vi "_debug_path_create.vi"(9 "Points":T1[](array[typedef]) {"RotationTarget"."rotation"."SIN" format="%13.4f"; "RotationTarget"."rotation"."COS" format="%13.4f"; "RotationTarget"."rotation"."VALUE" format="%13.4f"; "Position"."Y" format="%14.3f"; "Position"."X" format="%14.3f"}, 11 "file path":path) -> (1 "out Points":T1[](array[typedef]) {"RotationTarget"."rotation"."SIN" format="%13.4f"; "RotationTarget"."rotation"."COS" format="%13.4f"; "RotationTarget"."rotation"."VALUE" format="%13.4f"; "Position"."Y" format="%14.3f"; "Position"."X" format="%14.3f"})   [LabVIEW 2019]
uses:
  <vilib>/Rock Robotics/WPI/ThirdParty/MJansen/PathPlanner/TypeDef/PathPlannerPathPoint.ctl
  <vilib>/Rock Robotics/WPI/ThirdParty/JAS_Junk/TrajLib/TypeDef/TRANSLATION2D.ctl
  <vilib>/Rock Robotics/WPI/ThirdParty/MJansen/PathPlanner/TypeDef/PathPlannerPathConstraints.ctl
  <vilib>/Rock Robotics/WPI/ThirdParty/MJansen/PathPlanner/TypeDef/PathPlannerRotationTarget.ctl
  <vilib>/Rock Robotics/WPI/ThirdParty/JAS_Junk/TrajLib/TypeDef/ROTATION2D.ctl
  <vilib>/Rock Robotics/WPI/ThirdParty/JAS_Junk/TrajLib/Trajectory_Library.lvlib
  <vilib>/Rock Robotics/WPI/ThirdParty/MJansen/PathPlanner/PathPlanner24.lvlib
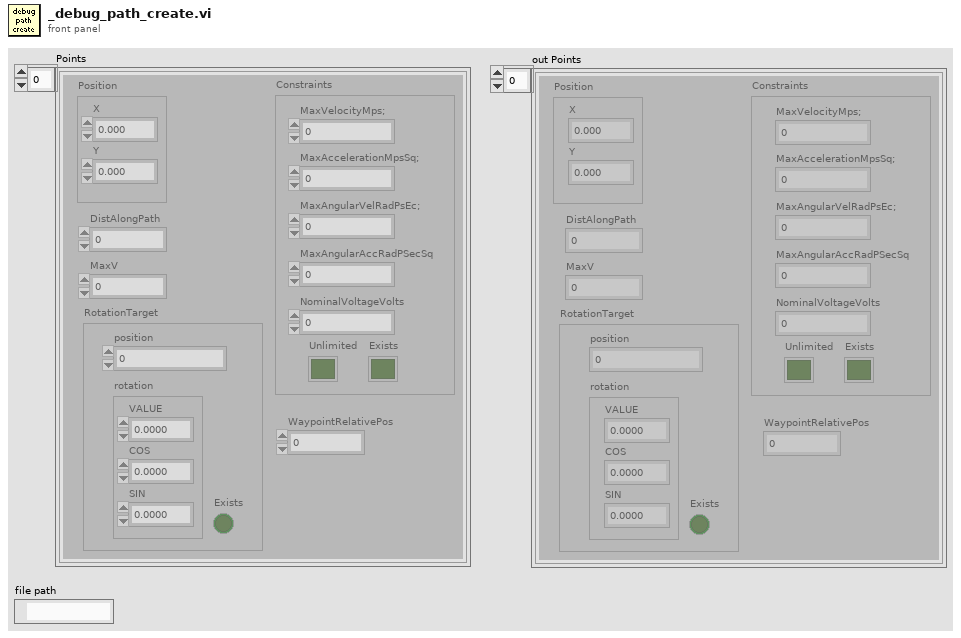
[diagram p1: front panel]
types:
  T1 = typedef "PathPlanner24.lvlib/PathPlannerPathPoint.ctl" = cluster{"Position":T2, "DistAlongPath":dbl, "MaxV":dbl, "Constraints":T3, "RotationTarget":T4, "WaypointRelativePos":dbl}
  T2 = typedef "Trajectory_Library.lvlib/TRANSLATION2D.ctl" = cluster{"X":dbl, "Y":dbl}
  T3 = typedef "PathPlanner24.lvlib/PathPlannerPathConstraints.ctl" = cluster{"MaxVelocityMps;":dbl, "MaxAccelerationMpsSq;":dbl, "MaxAngularVelRadPsEc;":dbl, "MaxAngularAccRadPSecSq":dbl, "Exists":bool, "Unlimited":bool, "NominalVoltageVolts":dbl}
  T4 = typedef "PathPlanner24.lvlib/PathPlannerRotationTarget.ctl" = cluster{"position":dbl, "rotation":T5, "Exists":bool}
  T5 = typedef "Trajectory_Library.lvlib/ROTATION2D.ctl" = cluster{"VALUE":dbl, "COS":dbl, "SIN":dbl}
  T6 = enum16{"open", "replace", "create", "open or create", "replace or create", "replace or create with confirmation"}
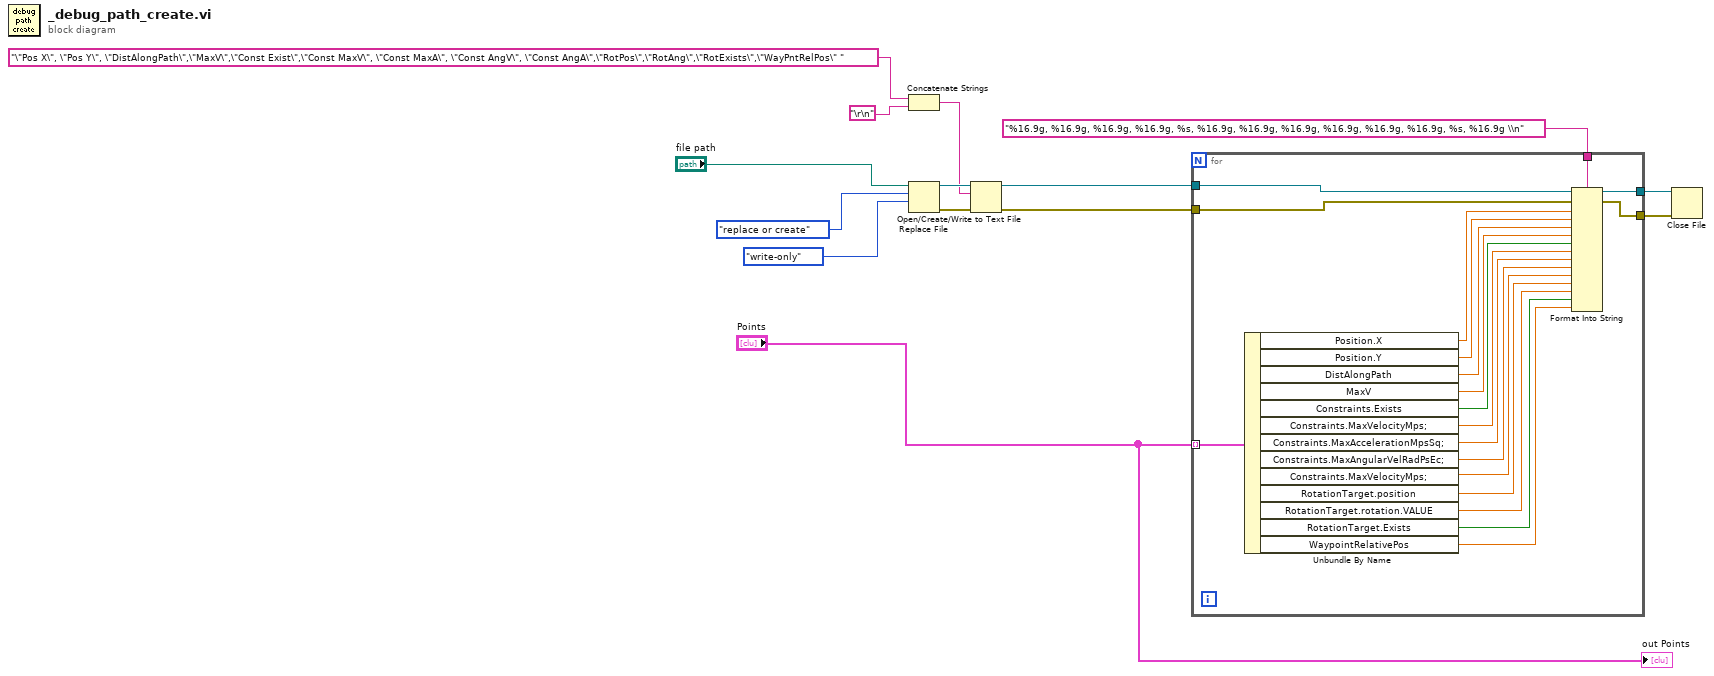
[diagram p0: block diagram]
diagram:
  n1 = Concatenate Strings("\"Pos X\", \"Pos Y\", \"DistAlongPath\",\"MaxV\",\"Const Exist\",\"Const MaxV\", \"Const MaxA\", \"Const AngV\", \"Const AngA\",\"RotPos\",\"RotAng\",\"RotExists\",\"WayPntRelPos\" " ("text"), "\r\n") -> (w7:string)
  n2 = Open/Create/Replace File(file path (use dialog)="file path", operation (0:open)=T6."replace or create", access (0:read/write)=enum16{"read/write", "read-only", "write-only"}."write-only") -> (refnum out=w11:refnum<file>, error out=w10:errorcluster)  [unwired: 3 in, 1 out]
  n3 = Write to Text File(file (use dialog)=w11, text=w7, error in=w10) -> (refnum out=w5:refnum<file>, error out=w6:errorcluster)  [unwired: 1 in, 1 out]
  n4 = for {
    tunnel: "Points" -> [w33] mode=indexing
    tunnel: w6 -> [w31]
    tunnel: w5 -> [w32]
    tunnel: [w30] -> w4
    tunnel: [w29] -> w3
    tunnel: "%16.9g, %16.9g, %16.9g, %16.9g, %s, %16.9g, %16.9g, %16.9g, %16.9g, %16.9g, %16.9g, %s, %16.9g \\n" ("format string") -> [w15]
    n5 = Unbundle By Name(w33) -> ("Position.X"=w28:dbl, "Position.Y"=w27:dbl, "DistAlongPath"=w26:dbl, "MaxV"=w25:dbl, "Constraints.Exists"=w24:bool, "Constraints.MaxVelocityMps;"=w23:dbl, "Constraints.MaxAccelerationMpsSq;"=w22:dbl, "Constraints.MaxAngularVelRadPsEc;"=w21:dbl, "Constraints.MaxVelocityMps;"=w20:dbl, "RotationTarget.position"=w19:dbl, "RotationTarget.rotation.VALUE"=w18:dbl, "RotationTarget.Exists"=w17:bool, "WaypointRelativePos"=w16:dbl)
    n6 = Format Into String(format string=w15, initial string=w32, error in=w31, w28, w27, w26, w25, w24, w23, w22, w21, w20, w19, w18, w17, w16) -> (resulting string=w30:refnum<file>, error out=w29:errorcluster)
  }
  n7 = Close File(refnum=w4, error in=w3) -> ()  [unwired: 2 out]
  "out Points" <- "Points"
